vi "NI 9211 Convert to Temperature (Calibrated).vi"(3 "Temperature Units (C)":u16(ring) items=["Celsius", "Fahrenheit", "Kelvin", "Rankine"], 4 "Autozero Channel":dbl, 5 "CJC Channel":dbl, 7 "Thermocouple Channel":dbl) -> (1 "Linearized Temperature":sgl format="%.6f")   [LabVIEW 2011]
doc: "Converts a fixed-point voltage read from a thermocouple into a temperature value."
panel:
  # "National Instruments has chosen thermocouple polynomial expressions that are valid only for  particular temperature ranges (given in the VI diagram).  These polynomials come from the NIST Monograph 175.\n\nIf you wish to use a different conversion formula, you can edit this VI and enter your own equation into the appropriate formula node."
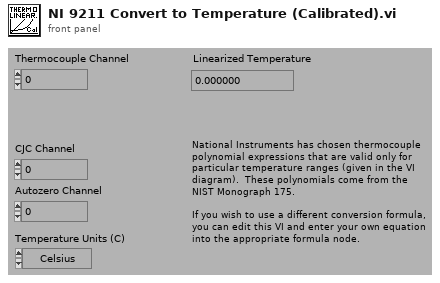
[diagram p1: front panel]
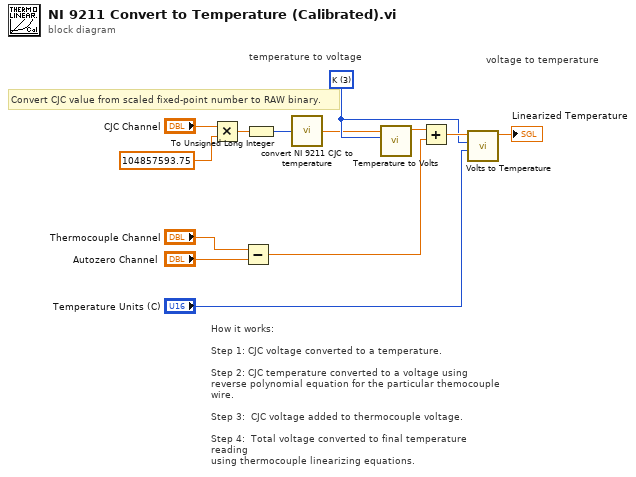
[diagram p0: block diagram]
diagram:
  w11 = u16 3 items=["B", "E", "J", "K", "R", "S", "T", "N", "IC (C)", "IC (F)", "Therm."] ("ThermocoupleType")
  # "Convert CJC value from scaled fixed-point number to RAW binary."
  # "How it works:\n\nStep 1: CJC voltage converted to a temperature.\n\nStep 2: CJC temperature converted to a voltage using reverse polynomial equation for the particular themocouple wire.\n\nStep 3:  CJC voltage added to thermocouple voltage.\n\nStep 4:  Total voltage converted to final temperature reading \nusing thermocouple linearizing equations."
  # "voltage to temperature"
  # "temperature to voltage"
  n1 = Multiply(x="CJC Channel", y=104857593.75) -> (x*y=w1:dbl)
  n2 = Subtract(x="Thermocouple Channel", y="Autozero Channel") -> (x-y=w4:dbl)
  n3 = To Unsigned Long Integer(number=w1) -> (unsigned 32bit integer=w5:u32)
  n4 = call "convert NI 9211 CJC to temperature.vi"("CJC Channel"=w5) -> ("CJC Temperature (C)"=w6:sgl)
  n5 = call "Temperature to Volts.vi"("ThermocoupleType"=w11, "Temperature"=w6) -> ("Thermocouple Voltage"=w13:sgl)  [unwired: 1 in, 4 out]
  n6 = Add(x=w13, y=w4) -> (x+y=w12:dbl)
  n7 = call "Volts to Temperature.vi"("Temperature Units"="Temperature Units (C)", "ThermocoupleType"=w11, "Thermocouple Voltage"=w12) -> ("Temperature"=→"Linearized Temperature":sgl)  [unwired: 4 out]
